vi "set channel data type.vi"(8 "error in (no error)":errorcluster, 9 "data type":i32, 10 "id":string, 11 "DSFConfiguration in":refnum<class "DSFConfiguration.lvclass">) -> (0 "error out":errorcluster, 3 "DSFConfiguration out":refnum<class "DSFConfiguration.lvclass">)   [LabVIEW 2017, in "DSFConfiguration.lvclass"]
uses:
  DSFConfiguration.lvclass
  DSFConfiguration.lvclass/DSFConfiguration.ctl
  DSFChannel/DSFChannel.lvclass/DSFChannel.ctl
  DSFChannel/Write data type.vi
  DSFChannel/DSFChannel.lvclass
  C:/github/data-sharing-framework/Source/Configuration API/Classes/IDable/IDable.lvclass
  <vilib>/Utility/error.llb/Error Cluster From Error Code.vi
  <vilib>/ErrorRing/Error Ring.xnode
  ID API/ID API.lvclass
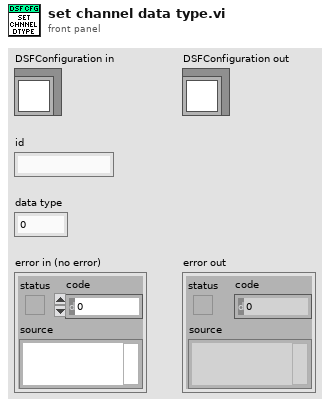
[diagram p1: front panel]
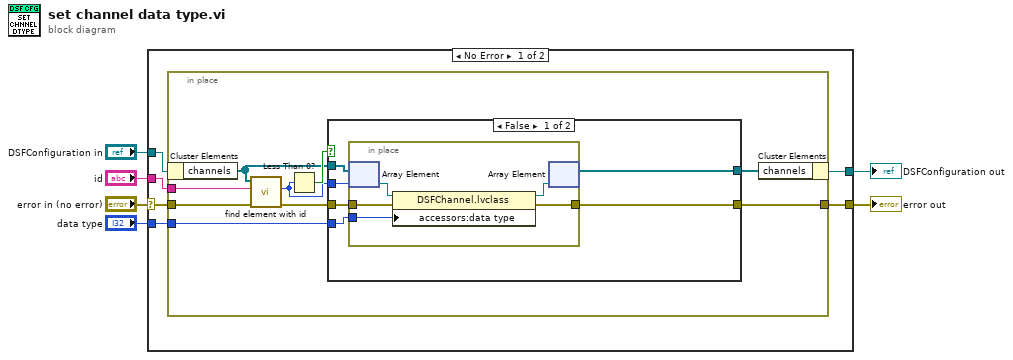
[diagram p0: block diagram]
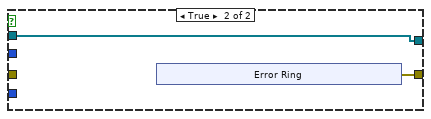
[diagram p2: hidden frame]
diagram:
  n1 = case shown="No Error" "error in (no error)" {
    selector: "error in (no error)" -> [w10 w40]
    tunnel: [w8 w40] -> w5
    tunnel: [w9 w39] -> w3
    tunnel: "DSFConfiguration in" -> [w12 w39]
    tunnel: "id" -> [w11 _]
    tunnel: "data type" -> [w7 _]
    frame No Error {
      n2 = in-place {
        in-place-border: w11 -> [w21]
        in-place-border: w10 -> [w20]
        in-place-border: [w17] -> w8
        in-place-border: w7 -> [w14]
        n3 = in-place-cluster #1(w12) -> ("channels"=w16:refnum<class "DSFChannel.lvclass">[])
        n4 = call "find element with id.vi"("error in (no error)"=w20, "id"=w21, "IDable Array in"=w16) -> ("error out"=w18:errorcluster, "index"=w15:i32)  [unwired: 7 in]
        n5 = Less Than 0?(x=w15) -> (x < 0?=w19:bool)
        n6 = case shown="False" w19 {
          tunnel: w18 -> [w24 _]
          tunnel: [w23 w34] -> w17
          tunnel: w16 -> [w27 w33]
          tunnel: w15 -> [w26 _]
          tunnel: w14 -> [w25 _]
          tunnel: [w22 w33] -> w13
          frame False {
            n7 = in-place {
              in-place-border: w25 -> [w31]
              in-place-border: w24 -> [w29]
              in-place-border: [w28] -> w23
              n8 = in-place-array #2(w27, w26) -> (w32:refnum<class "DSFChannel.lvclass">)
              n9 = property class="DSFChannel.lvclass"(reference=w32, error in=w29, "accessors:data type"=w31) -> (reference out=w30:refnum<class "DSFChannel.lvclass">, error out=w28:errorcluster)
              n10 = in-place-array #2(w30) -> (w22:refnum<class "DSFChannel.lvclass">[])  [unwired: 1 out]
            }
          }
          frame True {
            n11 = xnode "Error Ring"() -> ("error out"=w34:errorcluster)
          }
        }
        n12 = in-place-cluster #1("channels"=w13) -> (w9:refnum<class "DSFConfiguration.lvclass">)
      }
    }
    frame Error {
    }
  }
  "error out" <- w5
  "DSFConfiguration out" <- w3
